vi "MischerMonitor_set_Monitor_Values.vi"(4 "Mischer  Status":T1, 5 "System Monitor Variables (in)":T2) -> (1 "System Monitor Variables (out)":T2)   [LabVIEW 2019]
uses:
  Global/Global Variables/System Monitor Cluster.ctl
  Mischer/Mischer-Status.ctl
panel:
  # "2"
  # "to Condenser"
  # "1"
  # "7"
  # "From Still"
  # "5"
  # "Mischer\nEinheit"
  # "12"
  # "Cold\nTrap"
  # "Dump"
  # "9"
  # "8"
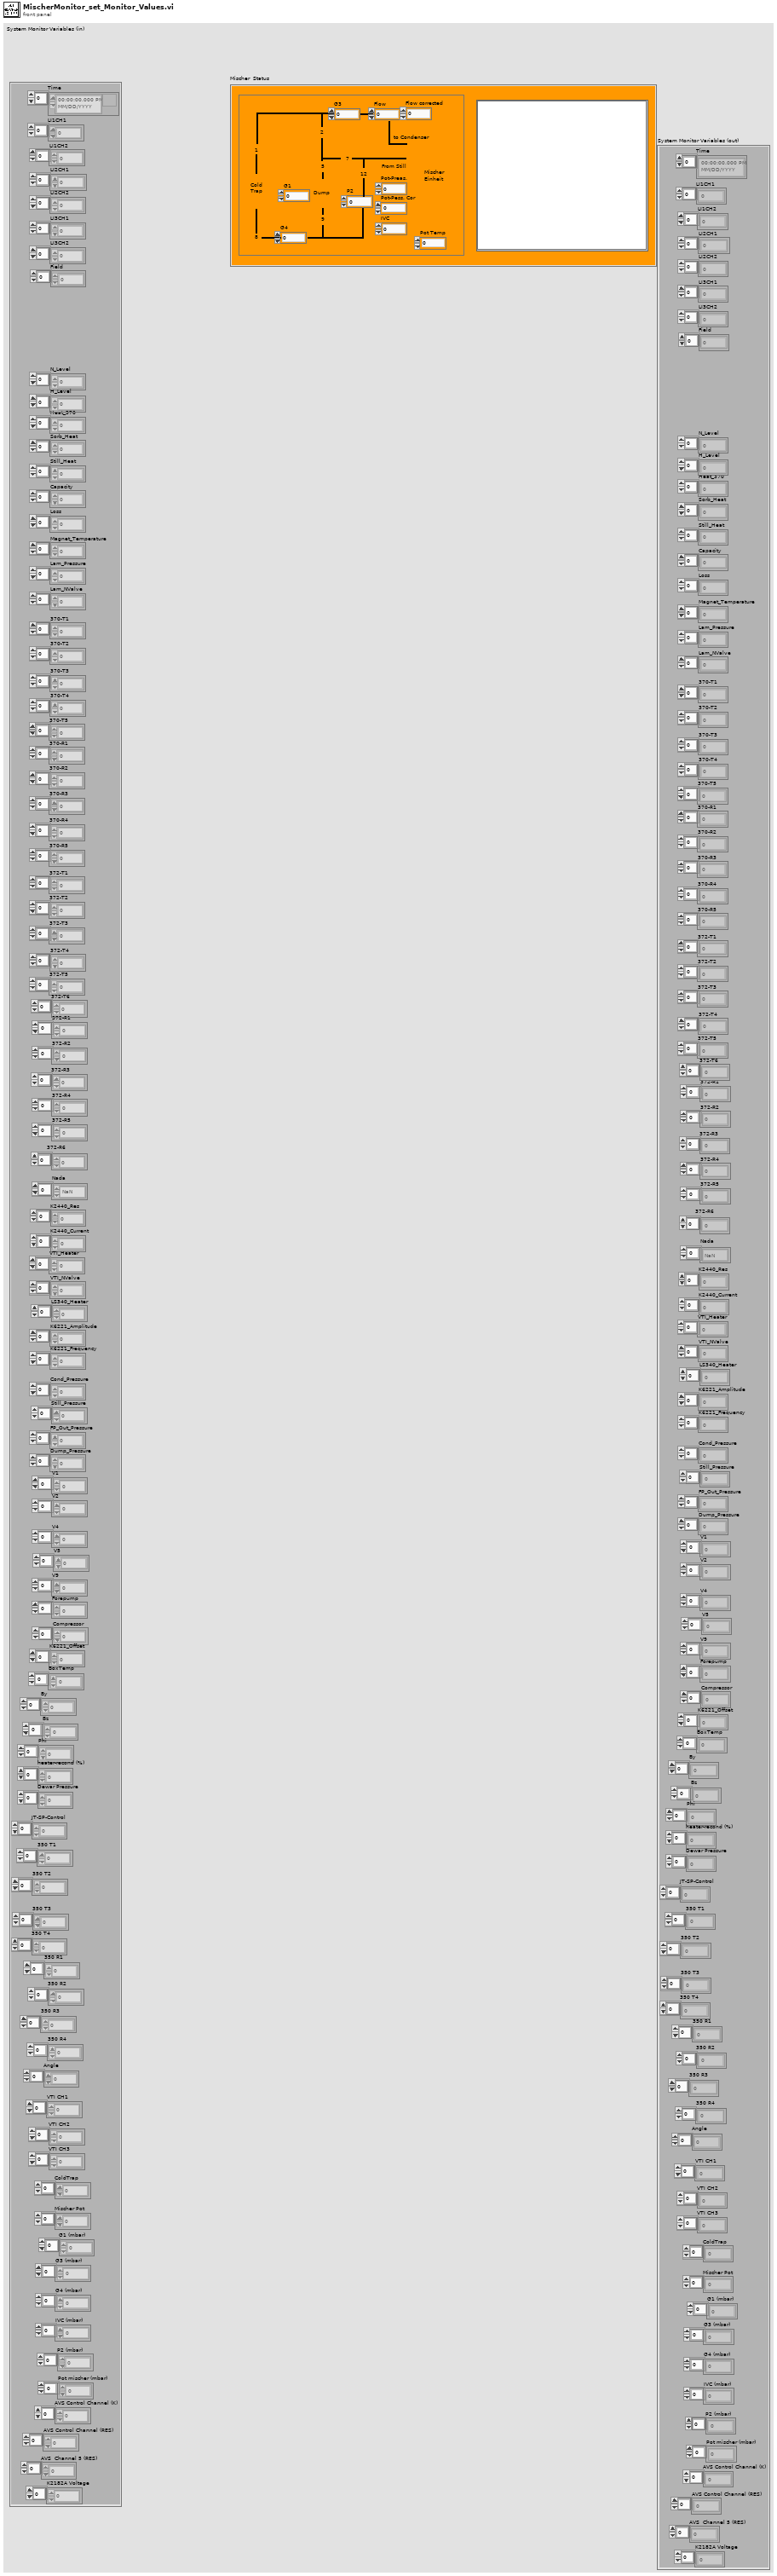
[diagram p1: front panel]
types:
  T1 = typedef "Mischer-Status.ctl" = cluster{"G4":dbl, "G1":dbl, "P2":dbl, "G3":dbl, "Flow":dbl, "Pot-Preas.":dbl, "IVC":dbl, "Flow corrected":dbl, "Pot-Pess. Cor":dbl, "Pot Temp":dbl, "Plot":dbl[][]}
  T2 = typedef "System Monitor Cluster.ctl" = cluster{"Time":timestamp[], "LI1CH1":dbl[], "LI1CH2":dbl[], "LI2CH1":dbl[], "LI2CH2":dbl[], "LI3CH1":dbl[], "LI3CH2":dbl[], "Field":dbl[], "N_Level":dbl[], "H_Level":dbl[], "Heat_370":dbl[], "Sorb_Heat":dbl[], "Still_Heat":dbl[], "Capacity":dbl[], "Loss":dbl[], "Magnet_Temperature":dbl[], "Lam_Pressure":dbl[], "Lam_NValve":dbl[], "370-T1":dbl[], "370-T2":dbl[], "370-T3":dbl[], "370-T4":dbl[], "370-T5":dbl[], "370-R1":dbl[], "370-R2":dbl[], "370-R3":dbl[], "370-R4":dbl[], "370-R5":dbl[], "372-T1":dbl[], "372-T2":dbl[], "372-T3":dbl[], "372-T4":dbl[], "372-T5":dbl[], "372-T6":dbl[], "372-R1":dbl[], "372-R2":dbl[], "372-R3":dbl[], "372-R4":dbl[], "372-R5":dbl[], "372-R6":dbl[], "Nada":dbl[], "K2440_Res":dbl[], "K2440_Current":dbl[], "VTI_Heater":dbl[], "VTI_NValve":dbl[], "LS340_Heater":dbl[], "K6221_Amplitude":dbl[], "K6221_Frequency":dbl[], "Cond_Pressure":dbl[], "Still_Pressure":dbl[], "FP_Out_Pressure":dbl[], "Dump_Pressure":dbl[], "V1":dbl[], "V2":dbl[], "V4":dbl[], "V5":dbl[], "V9":dbl[], "Forepump":dbl[], "Compressor":dbl[], "K6221_Offset":dbl[], "BoxTemp":dbl[], "By":dbl[], "Bz":dbl[], "Phi":dbl[], "heater-recond (%)":dbl[], "Dewar Pressure ":dbl[], "JT-SP-Control":dbl[], "350 T1":dbl[], "350 T2":dbl[], "350 T3":dbl[], "350 T4":dbl[], "350 R1":dbl[], "350 R2":dbl[], "350 R3":dbl[], "350 R4":dbl[], "Angle":dbl[], "VTI CH1":dbl[], "VTI CH2":dbl[], "VTI CH3":dbl[], "ColdTrap":dbl[], "Mischer Pot":dbl[], "G1 (mbar)":dbl[], "G3 (mbar) ":dbl[], "G4 (mbar)":dbl[], "IVC (mbar)":dbl[], "P2 (mbar) ":dbl[], "Pot mischer (mbar)":dbl[], "AVS Control Channel (K)":dbl[], "AVS Control Channel (RES)":dbl[], "AVS  Channel 5 (RES) ":dbl[], "K2182A Voltage":dbl[]}
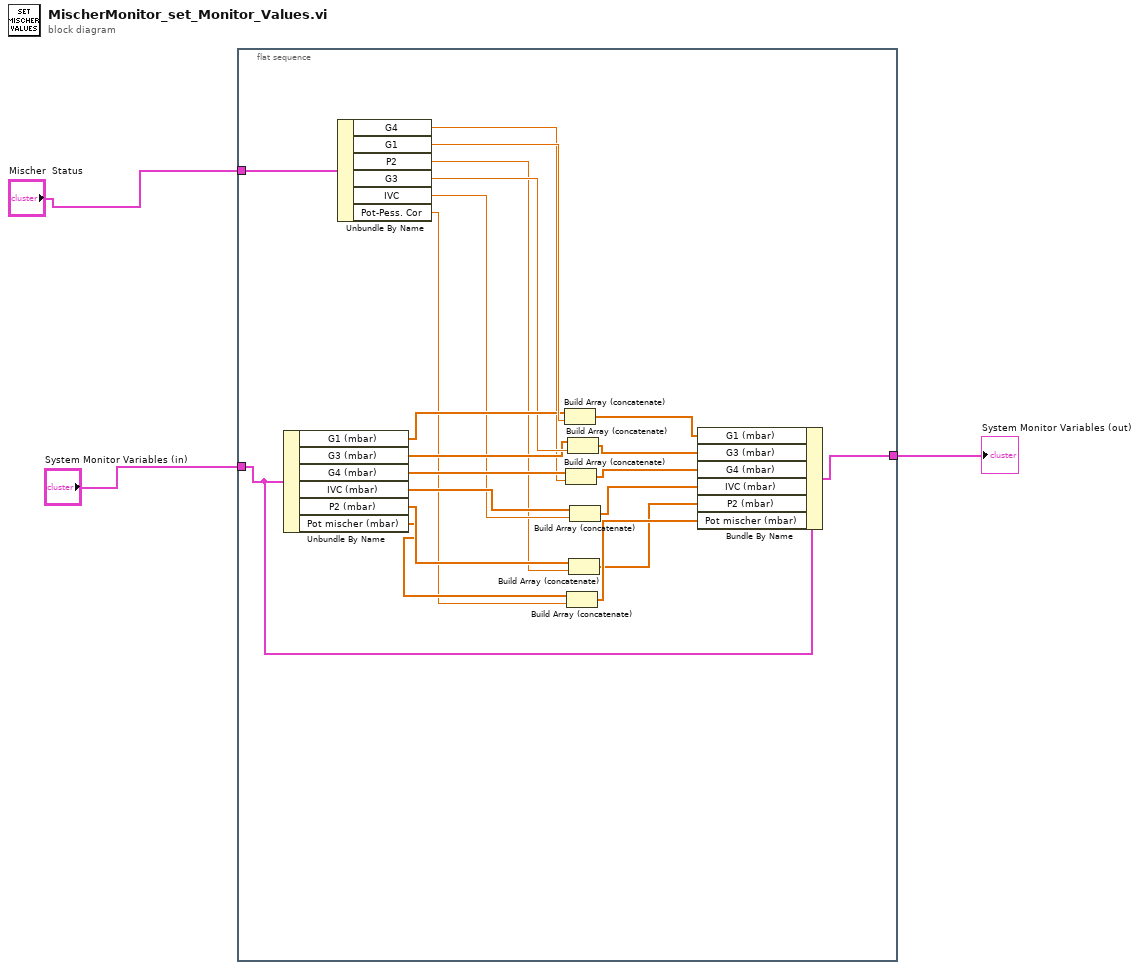
[diagram p0: block diagram]
diagram:
  n1 = flat-sequence {
    tunnel: "Mischer  Status" -> [w24]
    tunnel: "System Monitor Variables (in)" -> [w23]
    tunnel: [w22] -> w2
    frame #0 {
      n2 = Unbundle By Name(w23) -> ("G1 (mbar)"=w14:dbl[], "G3 (mbar)"=w12:dbl[], "G4 (mbar)"=w11:dbl[], "IVC (mbar)"=w9:dbl[], "P2 (mbar)"=w7:dbl[], "Pot mischer (mbar)"=w5:dbl[])
      n3 = Unbundle By Name(w24) -> ("G4"=w10:dbl, "G1"=w15:dbl, "P2"=w6:dbl, "G3"=w13:dbl, "IVC"=w8:dbl, "Pot-Pess. Cor"=w4:dbl)
      n4 = Build Array (concatenate)(w14, w15) -> (w21:dbl[])
      n5 = Build Array (concatenate)(w11, w10) -> (w19:dbl[])
      n6 = Build Array (concatenate)(w5, w4) -> (w18:dbl[])
      n7 = Build Array (concatenate)(w12, w13) -> (w20:dbl[])
      n8 = Build Array (concatenate)(w7, w6) -> (w17:dbl[])
      n9 = Build Array (concatenate)(w9, w8) -> (w16:dbl[])
      n10 = Bundle By Name(cluster=w23, "G1 (mbar)"=w21, "G3 (mbar)"=w20, "G4 (mbar)"=w19, "IVC (mbar)"=w16, "P2 (mbar)"=w17, "Pot mischer (mbar)"=w18) -> (w22:T2)
    }
  }
  "System Monitor Variables (out)" <- w2
